vi "Log Rx Map and Terminal Status.vi"(7 "Identifier":string, 9 "status lookup data":T9[](array[typedef]) {"terminal address" format="%.0x"; "remote terminal handle" format="%.0x"}, 10 "map from messages to value indexes":T1, 11 "log file":path=path "c:/ni-rt/VeriStand/Custom Devices/Initialize Rx EU.txt") -> ()   [LabVIEW 2020]
uses:
  Git/niveristand-ballard-milStd1553-custom-device/Source/Custom Device Support/Engine/Implementation/Rx Execution Unit/Status Terminal Lookup Data.ctl
  Git/niveristand-ballard-milStd1553-custom-device/Source/Custom Device Support/Shared/Map of Messages to Value Indexes.ctl
  Git/niveristand-ballard-milStd1553-custom-device/Source/Custom Device Support/Shared/Message Map Key.ctl
  Git/niveristand-ballard-milStd1553-custom-device/Source/Custom Device Support/Engine/Implementation/Rx Execution Unit/Message Map Value.ctl
  Git/niveristand-ballard-milStd1553-custom-device/Source/Custom Device Support/Shared/Message Definition.ctl
  Git/niveristand-ballard-milStd1553-custom-device/Source/Custom Device Support/Shared/Message Type.ctl
  Git/niveristand-ballard-milStd1553-custom-device/Source/Custom Device Support/Shared/Terminal Endpoint.ctl
  Git/niveristand-ballard-milStd1553-custom-device/Source/Custom Device Support/Shared/Address.ctl
  Git/niveristand-ballard-milStd1553-custom-device/Source/Custom Device Support/Shared/Parameter Definition.ctl
  Git/niveristand-ballard-milStd1553-custom-device/Source/Custom Device Support/Engine/Implementation/Rx Execution Unit/Rx Execution Unit.lvclass
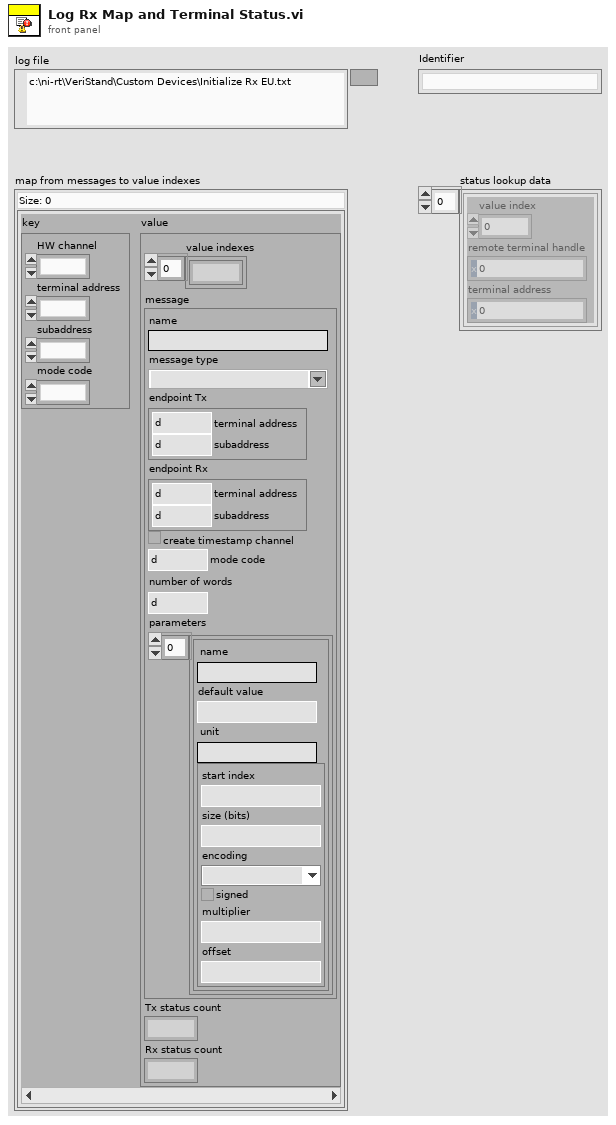
[diagram p1: front panel]
types:
  T1 = typedef "Map of Messages to Value Indexes.ctl" = map{T2, T3}
  T2 = typedef "Message Map Key.ctl" = cluster{"HW channel":u16, "terminal address":u16, "subaddress":u16, "mode code":u16}
  T3 = typedef "Ballard MIL-STD-1553 Engine.lvlib/Implementation.lvlib/Rx Execution Unit.lvclass/Message Map Value.ctl" = cluster{"value indexes":i32[], "message":T4, "Tx status count":i32, "Rx status count":i32}
  T4 = typedef "Message Definition.ctl" = cluster{"name":string, "message type":T5, "endpoint Tx":T6, "endpoint Rx":T6, "create timestamp channel":bool, "mode code":u16, "number of words":u16, "parameters":cluster{"name":string, "default value":dbl, "unit":string, "parameter definition":T8}[]}
  T5 = typedef "Message Type.ctl" = string
  T6 = typedef "Terminal Endpoint.ctl" = cluster{"terminal address":T7, "subaddress":T7}
  T7 = typedef "Address.ctl" = u16
  T8 = typedef "Parameter Definition.ctl" = cluster{"start index":i32, "size (bits)":i32, "encoding":enum16{"BNR", "BCD", "Discrete"}, "signed":bool, "multiplier":dbl, "offset":dbl}
  T9 = typedef "Ballard MIL-STD-1553 Engine.lvlib/Implementation.lvlib/Rx Execution Unit.lvclass/Status Terminal Lookup Data.ctl" = cluster{"value index":i32, "remote terminal handle":u64, "terminal address":u64}
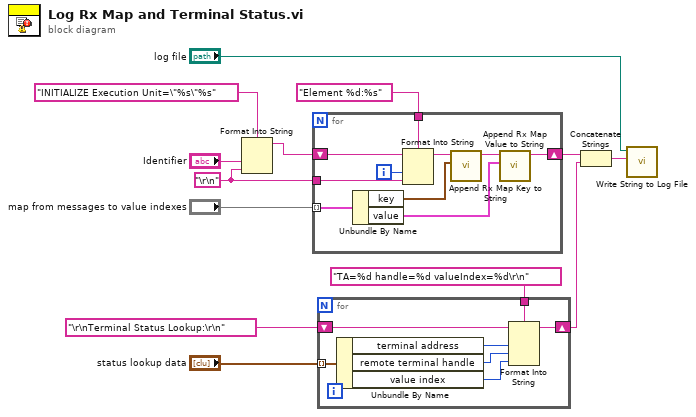
[diagram p0: block diagram]
diagram:
  w8 = "\r\n" ("format string")
  n1 = Format Into String(format string="INITIALIZE Execution Unit=\"%s\"%s", "Identifier", w8) -> (resulting string=w9:string)  [unwired: 2 in, 1 out]
  n2 = for {
    tunnel: "map from messages to value indexes" -> [w23] mode=indexing
    shift-right: [w14] -> w4
    shift-left: w9 -> [w20]
    tunnel: w8 -> [w18]
    tunnel: "Element %d:%s" ("format string") -> [w17]
    i -> [w19]
    n3 = Unbundle By Name(w23) -> ("key"=w22:T2, "value"=w21:T3)
    n4 = Format Into String(format string=w17, initial string=w20, w19, w18) -> (resulting string=w16:string)  [unwired: 1 in, 1 out]
    n5 = call "Append Rx Map Key to String.vi"("key"=w22, "String in"=w16) -> ("String out"=w15:string)  [unwired: 9 in]
    n6 = call "Append Rx Map Value to String.vi"("value"=w21, "String in"=w15) -> ("String"=w14:string)  [unwired: 9 in]
  }
  n7 = for {
    tunnel: "status lookup data" -> [w30] mode=indexing
    shift-right: [w25] -> w3
    shift-left: "\r\nTerminal Status Lookup:\r\n" ("format string") -> [w29]
    tunnel: "TA=%d handle=%d valueIndex=%d\r\n" ("format string") -> [w24]
    n8 = Unbundle By Name(w30) -> ("terminal address"=w28:u64, "remote terminal handle"=w27:u64, "value index"=w26:i32)
    n9 = Format Into String(format string=w24, initial string=w29, w28, w27, w26) -> (resulting string=w25:string)  [unwired: 1 in, 1 out]
  }
  n10 = Concatenate Strings(w4, w3) -> (w2:string)
  n11 = call "Write String to Log File.vi"("string to log"=w2, "log file"="log file") -> ()  [unwired: 9 in, 1 out]
